vi "Get_AxisArray.vi"(8 "error in (no error)":errorcluster, 10 "AxisArray":string[](array[string]), 11 "MotionModule configuration in":refnum<class "MotionModule configuration.lvclass">) -> (0 "error out":errorcluster, 3 "MotionModule configuration out":refnum<class "MotionModule configuration.lvclass">)   [LabVIEW 2017, in "MotionModule configuration.lvclass"]
uses:
  MotionModule configuration.lvclass
  MotionModule configuration.lvclass/MotionModule configuration.ctl
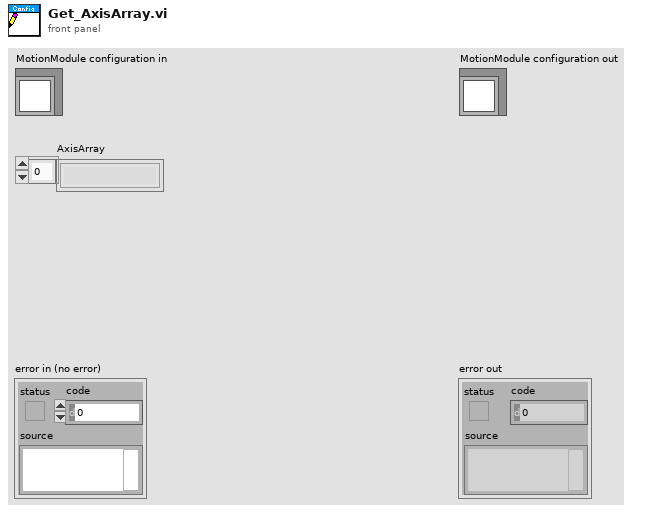
[diagram p1: front panel]
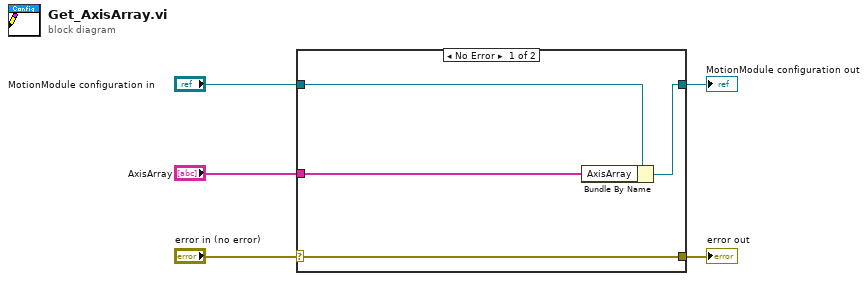
[diagram p0: block diagram]
diagram:
  n1 = case shown="No Error" "error in (no error)" {
    selector: "error in (no error)" -> [w9 w10]
    tunnel: [w9 w10] -> w4
    tunnel: [w7 w11] -> w2
    tunnel: "MotionModule configuration in" -> [w8 w11]
    tunnel: "AxisArray" -> [w6 _]
    frame No Error {
      n2 = Bundle By Name(cluster=w8, "AxisArray"=w6) -> (w7:refnum<class "MotionModule configuration.lvclass">)
    }
    frame Error {
    }
  }
  "error out" <- w4
  "MotionModule configuration out" <- w2
